vi "Configure AC Current.vi"(5 "Coupling (1: AC)":i32(ring)=1 items=["DC", "AC"], 6 "Filter (1:40 Hz)":i32(ring)=1 items=["100 Hz", "40 Hz", "10 Hz", "1 Hz"], 7 "Gate width (0: 50ms)":u16(ring) items=["50 ms", "1 s"], 8 "error in (no error)":errorcluster, 11 "VISA resource name":refnum<visa-resource-name>) -> (0 "error out":errorcluster, 3 "VISA resource name out":refnum<visa-resource-name>)   [LabVIEW 2011, in "Fluke 8508.lvlib"]
doc: "This VI sets AC Current specific settings such as the connection, filtering and conversion type on the instrument.\n\nNOTE: This VI does not have to be run just to set the instrument to make AC current measuremnts, but instead it is meant to be a supplement to the \"Configure Measurement\" VI which sets the measurement function, range, and resolution."
uses:
  Fluke 8508.lvlib
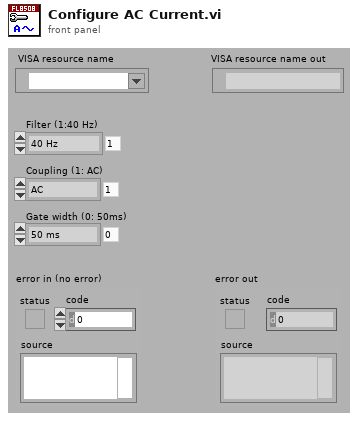
[diagram p1: front panel]
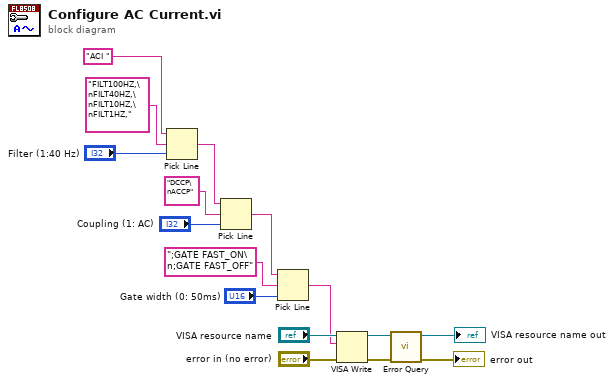
[diagram p0: block diagram]
diagram:
  n1 = Pick Line(string ("")="ACI ", multi-line string="FILT100HZ,\nFILT40HZ,\nFILT10HZ,\nFILT1HZ," ("true string"), line index="Filter (1:40 Hz)") -> (output string=w9:string)
  n2 = Pick Line(string ("")=w9, multi-line string="DCCP\nACCP", line index="Coupling (1: AC)") -> (output string=w1:string)
  n3 = Pick Line(string ("")=w1, multi-line string=";GATE FAST_ON\n;GATE FAST_OFF", line index="Gate width (0: 50ms)") -> (output string=w2:string)
  n4 = VISA Write(VISA resource name="VISA resource name", write buffer=w2, error in (no error)="error in (no error)") -> (VISA resource name out=w8:refnum<visa-resource-name>, error out=w7:errorcluster)  [unwired: 1 out]
  n5 = call "Error Query.vi"("error in (no error)"=w7, "VISA resource name"=w8) -> ("error out"=→"error out":errorcluster, "VISA resource name out"=→"VISA resource name out":refnum<visa-resource-name>)  [unwired: 6 in, 2 out]
